vi "From Variant.vi"(8 "Error In":errorcluster, 10 "Variant":variant, 11 "TD String In":refnum<class "String.lvclass">) -> (0 "Error Out":errorcluster, 3 "TD String Out":refnum<class "String.lvclass">)   [LabVIEW 2017, in "Tree API.lvlib" / "String.lvclass"]
doc: "Dynamic dispatch interface for conversion of variant LV data to Tree Data classes."
uses:
  String.lvclass
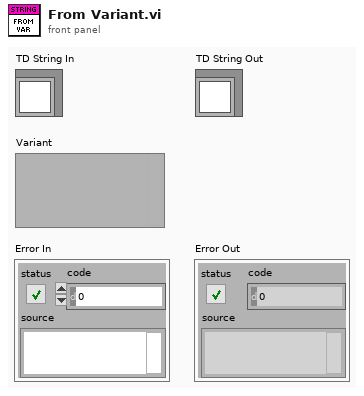
[diagram p1: front panel]
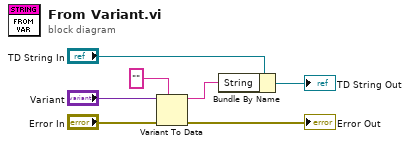
[diagram p0: block diagram]
diagram:
  n1 = Variant To Data(error in="Error In", type="" ("String Array"), Variant="Variant") -> (data=w3:string, error out=→"Error Out":errorcluster)
  n2 = Bundle By Name(cluster="TD String In", "String"=w3) -> (→"TD String Out":refnum<class "String.lvclass">)
